vi "TurretChooseAngle2.vi"(5 "Heading to Target Delta (best) [-180,+180]":dbl) -> (0 "Goal in Deadband":bool, 1 "Working Angular Delta":dbl)   [LabVIEW 2019]
panel:
  in  "Hysterisis":dbl
  in  "Current Turret Azimuth [0, 360]":dbl(knob)
  in  "Dead Zone Position B":dbl=100.0
  in  "Dead Zone Position A":dbl=80.0
  # "Counter Clock Wise = +\nClock Wise = -"
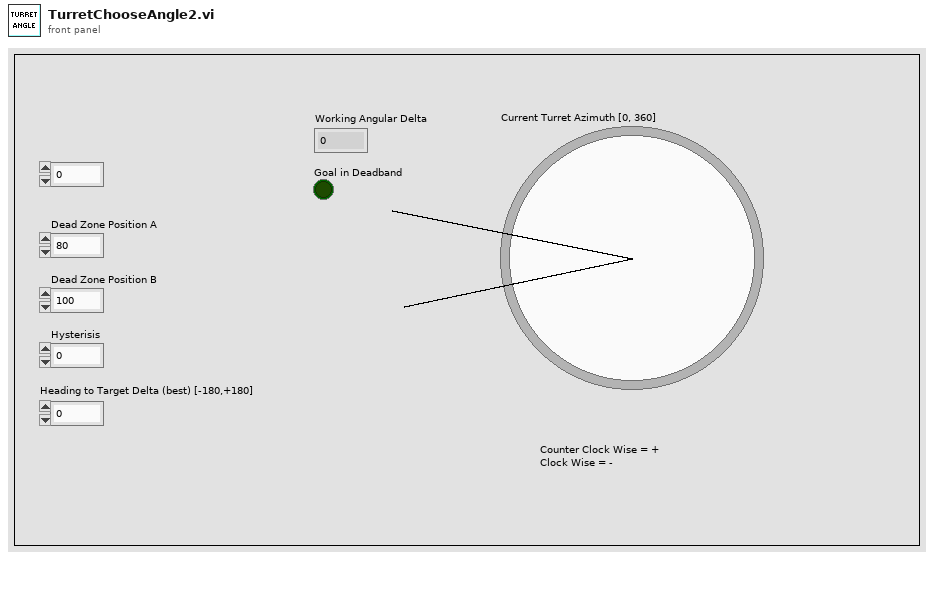
[diagram p1: front panel]
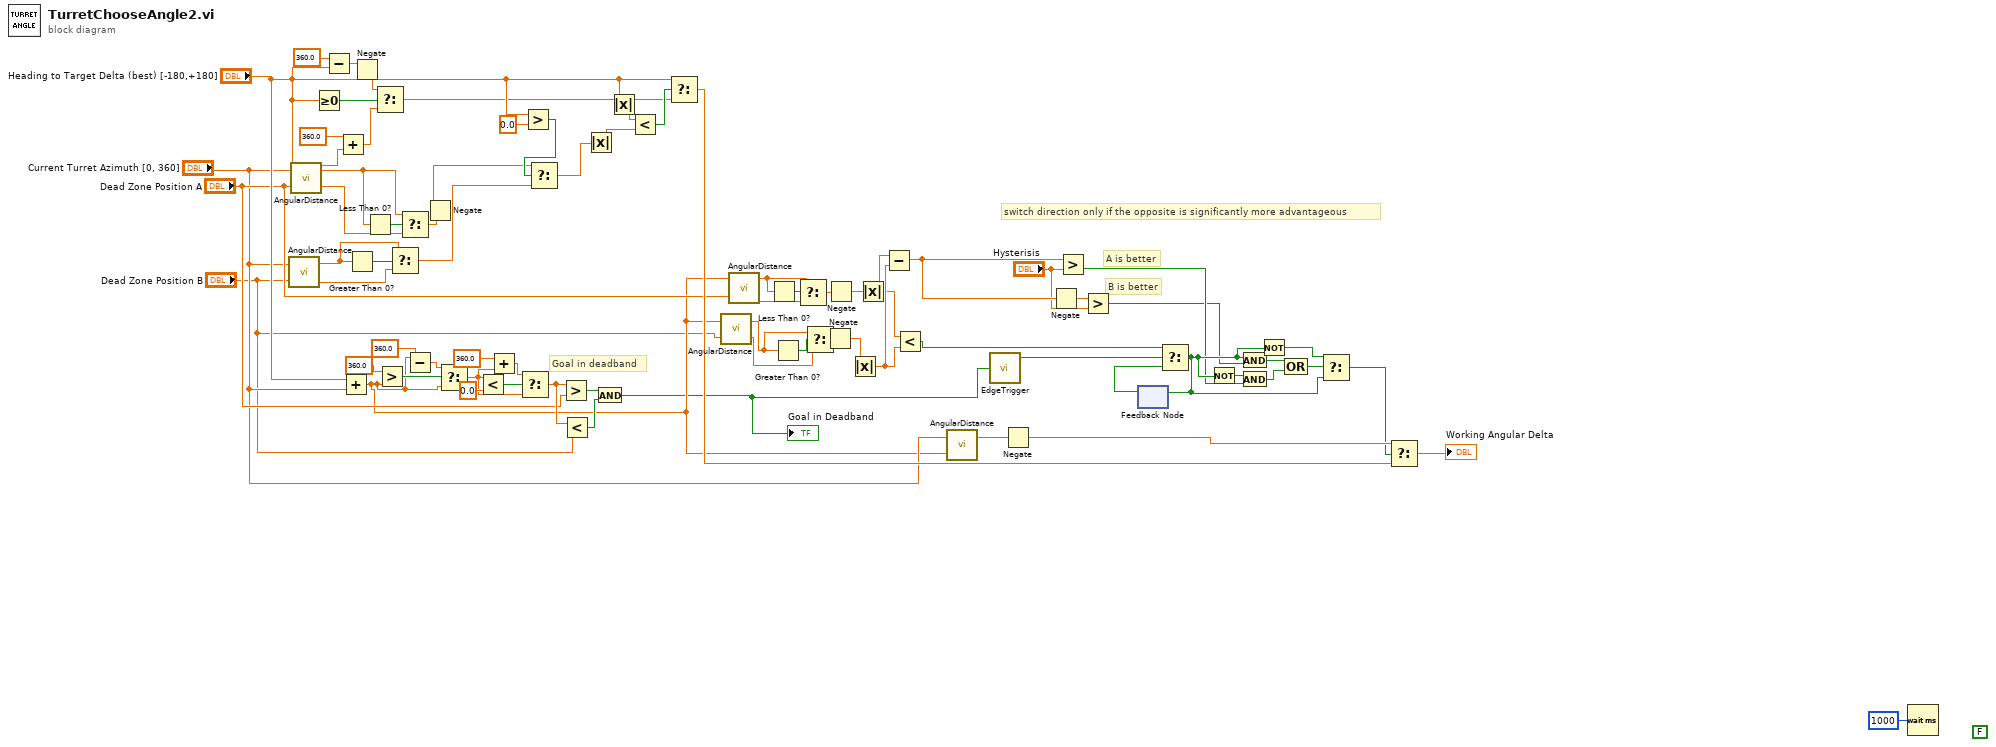
[diagram p0: block diagram]
diagram:
  (unwired) FALSE
  # "switch direction only if the opposite is significantly more advantageous"
  # "B is better"
  # "A is better"
  # "Goal in deadband"
  n1 = call "AngularDistance.vi"("Goal Angle (deg) [0,360]"="Dead Zone Position B", "Current Angle (deg) [-Inf,+Inf]"="Current Turret Azimuth [0, 360]") -> ("Alternate Signed Angular Distance (deg) [-180,+180]"=w70:dbl, "Signed Angular Distance (deg) [-180,+180]"=w71:dbl)
  n2 = call "AngularDistance.vi"("Goal Angle (deg) [0,360]"="Dead Zone Position A", "Current Angle (deg) [-Inf,+Inf]"="Current Turret Azimuth [0, 360]") -> ("Alternate Signed Angular Distance (deg) [-180,+180]"=w72:dbl, "Signed Angular Distance (deg) [-180,+180]"=w59:dbl)
  n3 = Greater Or Equal To 0?(x="Heading to Target Delta (best) [-180,+180]") -> (x >= 0?=w68:bool)
  n4 = Subtract(x=360.0, y="Heading to Target Delta (best) [-180,+180]") -> (x-y=w63:dbl)
  n5 = Add(x=360.0, y="Heading to Target Delta (best) [-180,+180]") -> (x+y=w61:dbl)
  n6 = Add(x="Heading to Target Delta (best) [-180,+180]", y="Current Turret Azimuth [0, 360]") -> (x+y=w31:dbl)
  n7 = Greater Than 0?(x=w71) -> (x > 0?=w55:bool)
  n8 = Negate(x=w63) -> (-x=w62:dbl)
  n9 = Less Than 0?(x=w59) -> (x < 0?=w56:bool)
  n10 = Select(t=w62, s=w68, f=w61) -> (s? t:f=w16:dbl)
  n11 = Greater?(x=360.0, y=w31) -> (0:w53:bool)
  n12 = Select(t=w71, s=w55, f=w70) -> (s? t:f=w17:dbl)
  n13 = Select(t=w59, s=w56, f=w72) -> (s? t:f=w66:dbl)
  n14 = Subtract(x=w31, y=360.0) -> (x-y=w51:dbl)
  n15 = Negate(x=w66) -> (-x=w18:dbl)
  n16 = Select(t=w51, s=w53, f=w31) -> (s? t:f=w46:dbl)
  n17 = Less?(x=w46, y=0.0) -> (x < y?=w49:bool)
  n18 = Add(x=360.0, y=w46) -> (x+y=w48:dbl)
  n19 = Select(t=w48, s=w49, f=w46) -> (s? t:f=w43:dbl)
  n20 = Greater?(x="Heading to Target Delta (best) [-180,+180]", y=0.0) -> (0:w57:bool)
  n21 = Select(t=w18, s=w57, f=w17) -> (s? t:f=w41:dbl)
  n22 = Greater?(x=w43, y="Dead Zone Position A") -> (0:w45:bool)
  n23 = Less?(x=w43, y="Dead Zone Position B") -> (x < y?=w44:bool)
  n24 = Absolute Value(x=w41) -> (abs(x)=w64:dbl)
  n25 = And(x=w45, y=w44) -> (x .and. y?=w11:bool)
  "Goal in Deadband" <- w11
  n26 = Absolute Value(x="Heading to Target Delta (best) [-180,+180]") -> (abs(x)=w65:dbl)
  n27 = Less?(x=w65, y=w64) -> (x < y?=w69:bool)
  n28 = Select(t="Heading to Target Delta (best) [-180,+180]", s=w69, f=w16) -> (s? t:f=w42:dbl)
  n29 = call "AngularDistance.vi"("Goal Angle (deg) [0,360]"="Dead Zone Position B", "Current Angle (deg) [-Inf,+Inf]"=w31) -> ("Alternate Signed Angular Distance (deg) [-180,+180]"=w22:dbl, "Signed Angular Distance (deg) [-180,+180]"=w23:dbl)
  n30 = call "AngularDistance.vi"("Goal Angle (deg) [0,360]"="Dead Zone Position A", "Current Angle (deg) [-Inf,+Inf]"=w31) -> ("Alternate Signed Angular Distance (deg) [-180,+180]"=w38:dbl, "Signed Angular Distance (deg) [-180,+180]"=w37:dbl)
  n31 = Less Than 0?(x=w37) -> (x < 0?=w36:bool)
  n32 = Greater Than 0?(x=w23) -> (x > 0?=w35:bool)
  n33 = Select(t=w37, s=w36, f=w38) -> (s? t:f=w25:dbl)
  n34 = Select(t=w23, s=w35, f=w22) -> (s? t:f=w24:dbl)
  n35 = Negate(x=w24) -> (-x=w20:dbl)
  n36 = Negate(x=w25) -> (-x=w19:dbl)
  n37 = Absolute Value(x=w20) -> (abs(x)=w28:dbl)
  n38 = Absolute Value(x=w19) -> (abs(x)=w27:dbl)
  n39 = Subtract(x=w27, y=w28) -> (x-y=w30:dbl)
  n40 = Less?(x=w27, y=w28) -> (x < y?=w12:bool)
  n41 = call "AngularDistance.vi"("Goal Angle (deg) [0,360]"=w31, "Current Angle (deg) [-Inf,+Inf]"="Current Turret Azimuth [0, 360]") -> ("Signed Angular Distance (deg) [-180,+180]"=w33:dbl)  [unwired: 1 out]
  n42 = call "EdgeTrigger.vi"("Input Signal"=w11) -> ("Rising Edge Trigger"=w13:bool)  [unwired: 2 out]
  n43 = Negate(x=w33) -> (-x=w39:dbl)
  n44 = Negate(x=w30) -> (-x=w29:dbl)
  n45 = Greater?(x=w30, y="Hysterisis") -> (0:w3:bool)
  n46 = Greater?(x=w29, y="Hysterisis") -> (0:w2:bool)
  n47 = feedback #1() -> (w14:bool)  [unwired: 1 in]
  n48 = Select(t=w12, s=w13, f=w14) -> (s? t:f=w6:bool)
  n49 = feedback-in #1(w6) -> ()
  n50 = Not(x=w6) -> (.not. x?=w8:bool)
  n51 = And(x=w6, y=w2) -> (x .and. y?=w10:bool)
  n52 = And(x=w8, y=w3) -> (x .and. y?=w9:bool)
  n53 = Not(x=w6) -> (.not. x?=w5:bool)
  n54 = Compound Arithmetic op=OR(w10, w9) -> (w7:bool)
  n55 = Select(t=w5, s=w7, f=w6) -> (s? t:f=w4:bool)
  n56 = Select(t=w39, s=w4, f=w42) -> (s? t:f=→"Working Angular Delta":dbl)
  n57 = Wait (ms)(milliseconds to wait=u32 1000) -> ()  [unwired: 1 out]
